vi "Build plots.vi"(9 "Im":dbl[](array[numeric]), 10 "Re":dbl[](array[numeric]), 11 "X":dbl[](array[numeric])) -> (3 "Plot_data":cluster{"Array":dbl[], "Im":dbl[]}[](array[cluster]))   [LabVIEW 2021]
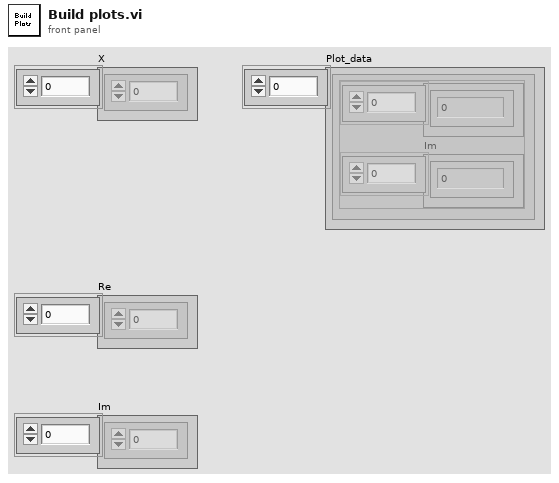
[diagram p1: front panel]
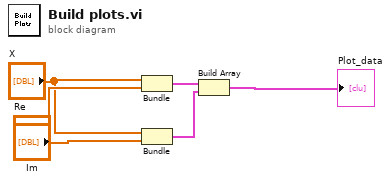
[diagram p0: block diagram]
diagram:
  n1 = Bundle("X"="X", "Re"="Re") -> (w1:cluster{"X":dbl[], "Re":dbl[]})  [unwired: 1 in]
  n2 = Bundle("X"="X", "Im"="Im") -> (w2:cluster{"X":dbl[], "Im":dbl[]})  [unwired: 1 in]
  n3 = Build Array(w1, w2) -> (→"Plot_data":cluster{"X":dbl[], "Im":dbl[]}[])
